vi "Create info string sub.vi"(0 "Sig gen waveform":string, 5 "Excitation laser OD":string="2.05", 7 "AM Rate (Hz)":dbl, 9 "AM Depth (%)":dbl, 11 "DAQ Rate (Hz)":dbl, 12 "Amplitude Modulation On?":bool, 13 "Amplitude (dBm)":dbl, 14 "Step Dwell (ms)":dbl) -> (4 "Info header":string)   [LabVIEW 2014]
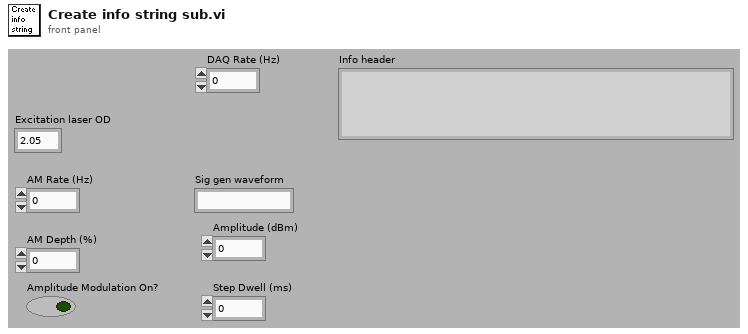
[diagram p1: front panel]
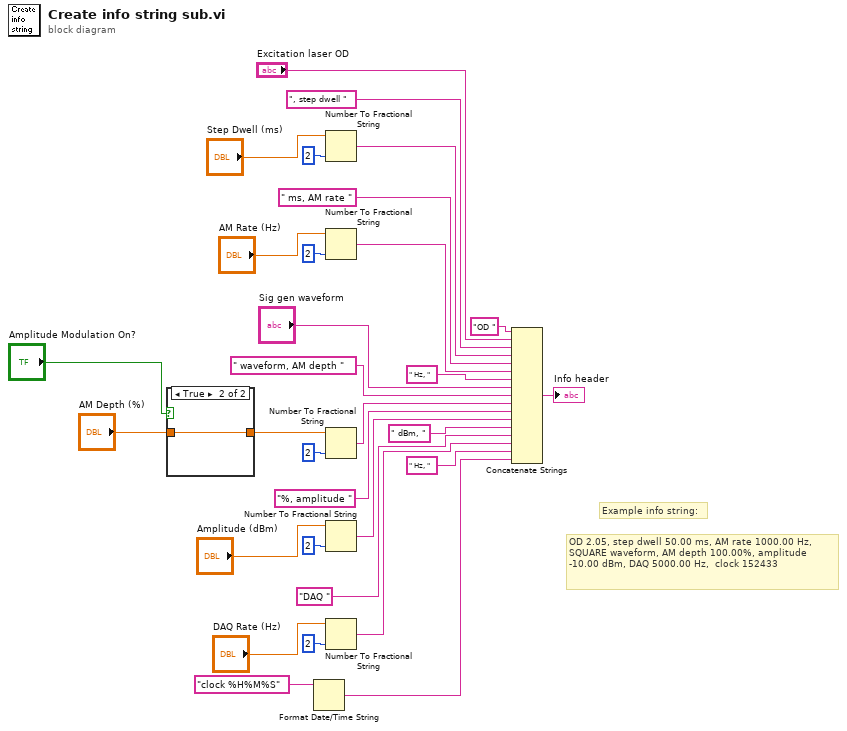
[diagram p0: block diagram]
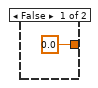
[diagram p2: hidden frame]
diagram:
  # "OD 2.05, step dwell 50.00 ms, AM rate 1000.00 Hz, SQUARE waveform, AM depth 100.00%, amplitude -10.00 dBm, DAQ 5000.00 Hz,  clock 152433"
  # "Example info string:"
  n1 = case shown="True" "Amplitude Modulation On?" {
    tunnel: [0.0 ("AM Depth (%)") w33] -> w29
    tunnel: "AM Depth (%)" -> [_ w33]
    frame False {
    }
    frame True {
    }
  }
  n2 = Format Date/Time String(time format string (%c)="clock %H%M%S") -> (date/time string=w1:string)  [unwired: 2 in]
  n3 = Number To Fractional String(number="Step Dwell (ms)", precision (6)=i16 2) -> (F-format string=w17:string)  [unwired: 2 in]
  n4 = Number To Fractional String(number="AM Rate (Hz)", precision (6)=i16 2) -> (F-format string=w19:string)  [unwired: 2 in]
  n5 = Number To Fractional String(number=w29, precision (6)=i16 2) -> (F-format string=w23:string)  [unwired: 2 in]
  n6 = Number To Fractional String(number="Amplitude (dBm)", precision (6)=i16 2) -> (F-format string=w25:string)  [unwired: 2 in]
  n7 = Number To Fractional String(number="DAQ Rate (Hz)", precision (6)=i16 2) -> (F-format string=w3:string)  [unwired: 2 in]
  n8 = Concatenate Strings("OD ", "Excitation laser OD", ", step dwell ", w17, " ms, AM rate ", w19, " Hz, ", "Sig gen waveform", " waveform, AM depth ", w23, "%, amplitude ", w25, " dBm, ", "DAQ ", w3, " Hz, ", w1) -> (→"Info header":string)
